vi "Generate Firmware Interface Config Message.vi"(8 "Error In":errorcluster, 9 "Firmware Program Interface Index":i32, 10 "Device Index":i32, 11 "Family Index":i32) -> (0 "Error Out":errorcluster, 3 "Config Message":string)   [LabVIEW 2011, in "LVH-LINX.lvlib"]
uses:
  LVH-LINX.lvlib
  Type Defs/All Firmware Data FGV States.ctl
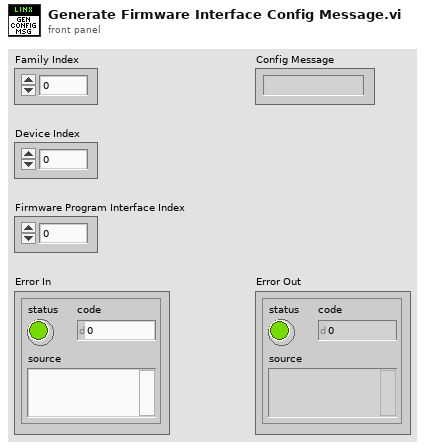
[diagram p1: front panel]
types:
  T1 = typedef "LVH-LINX.lvlib/All Firmware Data FGV States.ctl" = enum16{"Set", "Get"}
  T2 = typedef "LVH-LINX.lvlib/Device Data.ctl" = cluster{"Family ID":i32, "Family Name":string, "Device ID":i32, "Device Name":string, "Firmware Program Interfaces":string[], "Path":path}
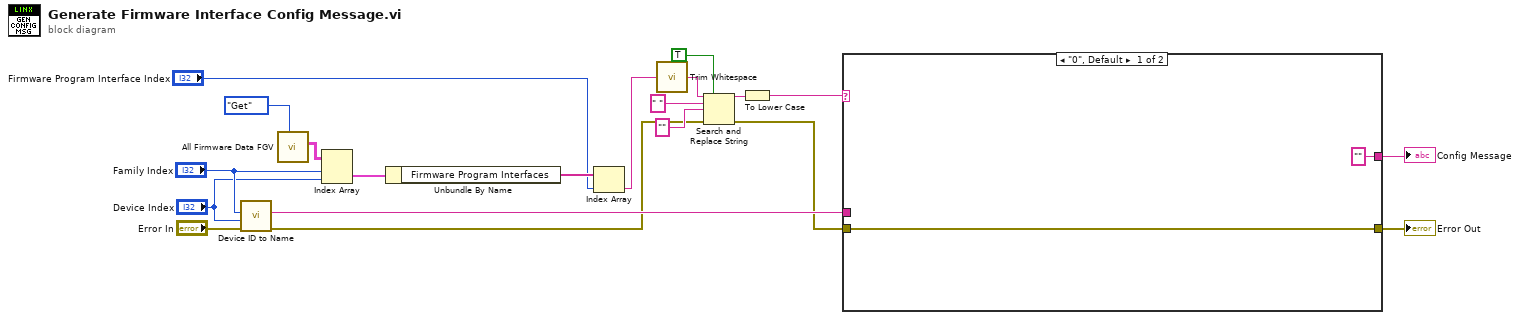
[diagram p0: block diagram]
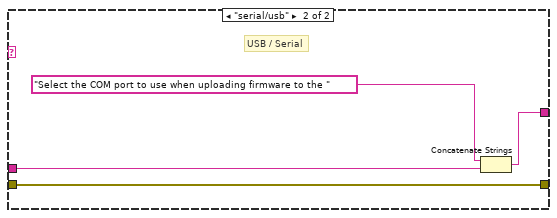
[diagram p2: hidden frame]
diagram:
  n1 = call "Device ID to Name.vi"("Error In"="Error In", "Device Index"="Device Index", "Family Index"="Family Index") -> ("Error Out"=w13:errorcluster, "Device Name"=w17:string)  [unwired: 6 in, 1 out]
  n2 = call "All Firmware Data FGV.vi"("All Firmware Data FGV States"=All_Firmware_Data_FGV_States."Get") -> ("Devices"=w11:T2[][])  [unwired: 7 in, 3 out]
  n3 = Index Array(array=w11, index (row)="Family Index", index (col)="Device Index") -> (element=w7:T2)
  n4 = Unbundle By Name(w7) -> ("Firmware Program Interfaces"=w6:string[])
  n5 = Index Array(array=w6, index="Firmware Program Interface Index") -> (element=w4:string)
  n6 = call <vilib>:"Trim Whitespace.vi"("string"=w4) -> ("trimmed string"=w16:string)  [unwired: 1 in]
  n7 = Search and Replace String(replace all?=TRUE ("replace all? (F)"), input string=w16, search string=" ", replace string="" ("replace string (\"\")"), error in=w13) -> (result string=w2:string, error out=w12:errorcluster)  [unwired: 3 in, 2 out]
  n8 = To Lower Case(string=w2) -> (all lower case string=w1:string)
  n9 = case shown="\"0\", Default" w1 {
    tunnel: w12 -> [w22 w24]
    tunnel: [w22 w24] -> w20
    tunnel: ["" w25] -> w19
    tunnel: w17 -> [_ w23]
    frame "0", Default {
    }
    frame "serial/usb" {
      # "USB / Serial"
      n10 = Concatenate Strings("Select the COM port to use when uploading firmware to the ", w23) -> (w25:string)
    }
  }
  "Error Out" <- w20
  "Config Message" <- w19
